vi "ControlMotorFindZero.vi"(6 "消息引用":refnum<vi>, 8 "错误输入（无错误）":errorcluster) -> (0 "错误输出":errorcluster)   [LabVIEW 2018]
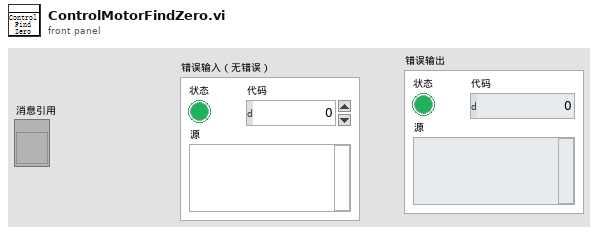
[diagram p1: front panel]
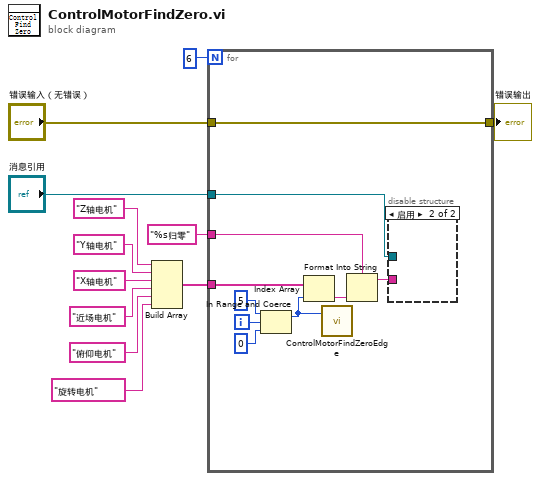
[diagram p0: block diagram]
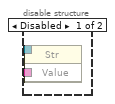
[diagram p2: hidden frame]
diagram:
  n1 = Build Array("Z轴电机", "Y轴电机", "X轴电机", "近场电机", "俯仰电机", "旋转电机") -> (w6:string[])
  n2 = for {
    N: 6 -> [_]
    tunnel: w6 -> [w22]
    tunnel: "消息引用" -> [w19]
    tunnel: "%s归零" ("格式字符串") -> [w17]
    tunnel: "错误输入（无错误）" -> [w13]
    tunnel: [w13] -> w1
    i -> [w15]
    n3 = In Range and Coerce(upper limit=5 ("上限"), x=w15, lower limit=0 ("下限")) -> (coerced(x)=w14:i32)  [unwired: 1 out]
    n4 = Index Array(array=w22, index=w14) -> (element=w18:string)
    n5 = call "ControlMotorFindZeroEdge.vi"("控制电机"=w14) -> ()  [unwired: 2 in]
    n6 = Format Into String(format string=w17, w18) -> (resulting string=w16:string)  [unwired: 2 in, 1 out]
    n7 = disable-structure shown="启用" {
      disable-tunnel: w19 -> [w24 _]
      disable-tunnel: w16 -> [w23 _]
      frame Disabled {
        n8 = property class="Str"(reference=w24, "Value"=w23) -> ()  [unwired: 1 in, 2 out]
      }
      frame Enabled {
      }
    }
  }
  "错误输出" <- w1
